vi "Fetch Multi Eval Meas List Segment Modulation Detected Allocation Results.vi"(8 "error in (no error)":errorcluster, 9 "Segment (1)":T3=1, 10 "Instance (1)":T4=1, 11 "VISA resource name":refnum<visa-resource-name>) -> (0 "error out":errorcluster, 1 "Detected Allocation":T1, 2 "Reliability":T2, 3 "VISA resource name out":refnum<visa-resource-name>)   [LabVIEW 2020, in "Rohde&Schwarz CMWXP NR FR1 Measurement.lvlib"]
doc: "Return the detected allocation for segment <no> in list mode.\n\nThe result is determined from the last measured slot of the statistical length. The individual measurements provide identical detected allocation results when measuring the same slot. However, different statistical lengths can be defined for the measurements so that the measured slots and returned results can differ.\n\nAttribute:\nRSCMWXPNRFR1M_ATTR_FETCH_MULTI_EVAL_MEAS_LIST_SEGMENT_MODULATION_DETECTED_ALLOCATION_RESULTS\n\nRemote-control command:\nFETCh:NRSub:MEAS<i>:MEValuation:LIST:SEGMent<no>:MODulation:DALLocation?"
uses:
  <instrlib>/Rohde&Schwarz CMWXP NR FR1 Measurement/Rohde&Schwarz CMWXP NR FR1 Measurement.lvlib
  <instrlib>/Rohde&Schwarz CMWXP NR FR1 Measurement/Private/_Instance.ctl
  <instrlib>/Rohde&Schwarz CMWXP NR FR1 Measurement/Private/_Segment.ctl
  <instrlib>/Rohde&Schwarz CMWXP NR FR1 Measurement/Private/_SegReliability.ctl
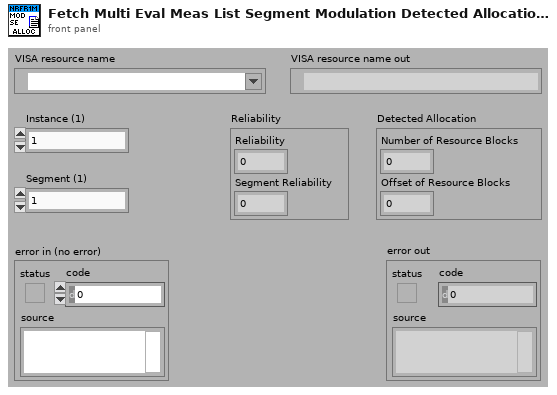
[diagram p1: front panel]
types:
  T1 = cluster{"Number of Resource Blocks":i32, "Offset of Resource Blocks":i32}
  T2 = typedef "Rohde&Schwarz CMWXP NR FR1 Measurement.lvlib/_SegReliability.ctl" = cluster{"Reliability":i32, "Segment Reliability":i32}
  T3 = typedef "Rohde&Schwarz CMWXP NR FR1 Measurement.lvlib/_Segment.ctl" = i32
  T4 = typedef "Rohde&Schwarz CMWXP NR FR1 Measurement.lvlib/_Instance.ctl" = i32
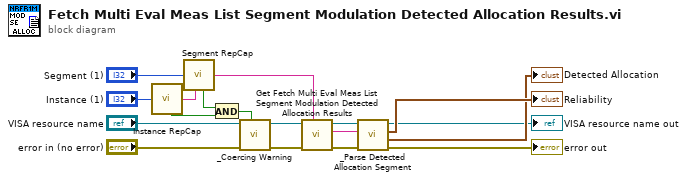
[diagram p0: block diagram]
diagram:
  n1 = call <instrlib>:"Instance RepCap.vi"("Instance In"="Instance (1)") -> ("In Range?"=w13:bool, "RepCap Identifier Out"=w12:string)  [unwired: 1 in]
  n2 = call <instrlib>:"Segment RepCap.vi"("Segment In"="Segment (1)", "RepCap String In (\"\")"=w12) -> ("In Range?"=w11:bool, "RepCap Identifier Out"=w10:string)
  n3 = And(x=w11, y=w13) -> (x .and. y?=w14:bool)
  n4 = call <instrlib>:"_Coercing Warning.vi"("In Range?"=w14, "error in (no error)"="error in (no error)", "VISA resource name"="VISA resource name") -> ("error out"=w8:errorcluster, "VISA resource name out"=w9:refnum<visa-resource-name>)  [unwired: 7 in]
  n5 = call "Get Fetch Multi Eval Meas List Segment Modulation Detected Allocation Results"("Repeated Capabilities"=w10, "error in (no error)"=w8, "instrument handle"=w9) -> ("error out"=w5:errorcluster, "Fetch Multi Eval Meas List Segment Modulation Detected Allocation Results"=w6:string, "instrument handle out"=w7:refnum<visa-resource-name>)  [unwired: 6 in]
  n6 = call <instrlib>:"_Parse Detected Allocation Segment.vi"("error in (no error)"=w5, "Input String"=w6, "VISA resource name"=w7) -> ("error out"=→"error out":errorcluster, "Detected Allocation"=→"Detected Allocation":T1, "Reliability Results"=→"Reliability":T2, "VISA resource name out"=→"VISA resource name out":refnum<visa-resource-name>)  [unwired: 5 in]
